vi "3.1.vi"() -> ()   [LabVIEW 2020]
panel:
  out "Grafica":cluster{dbl, dbl, dbl}[](graph)
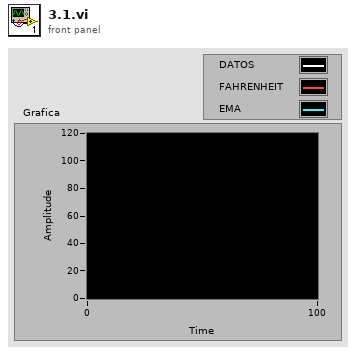
[diagram p1: front panel]
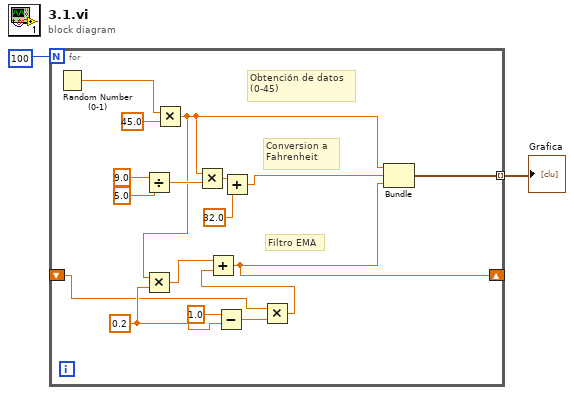
[diagram p0: block diagram]
diagram:
  n1 = for {
    N: 100 -> [_]
    shift-right: [w5] -> _
    shift-left: _ -> [w6]
    tunnel: [w3] -> w1 mode=indexing
    w9 = 0.2 ("y")
    # "Filtro EMA"
    # "Conversion a \nFahrenheit"
    # "Obtención de datos\n(0-45)"
    n2 = Random Number (0-1)() -> (number: 0 to 1=w19:dbl)
    n3 = Divide(x=9.0, y=5.0) -> (x/y=w17:dbl)
    n4 = Multiply(x=w19, y=45.0) -> (x*y=w7:dbl)
    n5 = Multiply(x=w7, y=w9) -> (x*y=w12:dbl)
    n6 = Multiply(x=w7, y=w17) -> (x*y=w14:dbl)
    n7 = Subtract(x=1.0, y=w9) -> (x-y=w10:dbl)
    n8 = Add(x=w14, y=32.0) -> (x+y=w4:dbl)
    n9 = Multiply(x=w6, y=w10) -> (x*y=w11:dbl)
    n10 = Add(x=w12, y=w11) -> (x+y=w5:dbl)
    n11 = Bundle(w7, w4, w5) -> (w3:cluster{dbl, dbl, dbl})  [unwired: 1 in]
  }
  "Grafica" <- w1
